vi "Configure Power Analysis (Modulation).vi"(8 "error in (no error)":errorcluster, 9 "Measurement Type (4: Frequency)":i32(ring)=4 items=["Vaverage", "Acrms", "Vratio", "Period", "Frequency", "Pwidth", "Nwidth", "Duty Cycle", "Rise Time", "Fall Time"], 10 "Source (0: V)":i32(ring) items=["V", "I"], 11 "VISA resource name":refnum<visa-resource-name>) -> (0 "error out":errorcluster, 3 "VISA resource name out":refnum<visa-resource-name>)   [LabVIEW 2016, in "Agilent 2000 3000 X-Series.lvlib"]
doc: "Applies a specific modulation analysis type.\n\n<B>Note(s):</B>\nThe Modulation analysis measures the control pulse signal to a switching device (MOSFET) and observes the trending of the pulse width, duty cycle, period, frequency, etc. of the control pulse signal.\n\nUse <B>Read Measurement (Static).vi</B> to read the result of this power analysis."
uses:
  Agilent 2000 3000 X-Series.lvlib
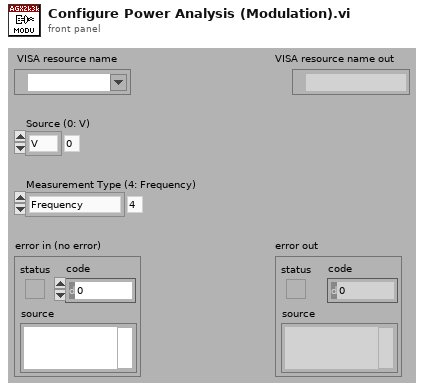
[diagram p1: front panel]
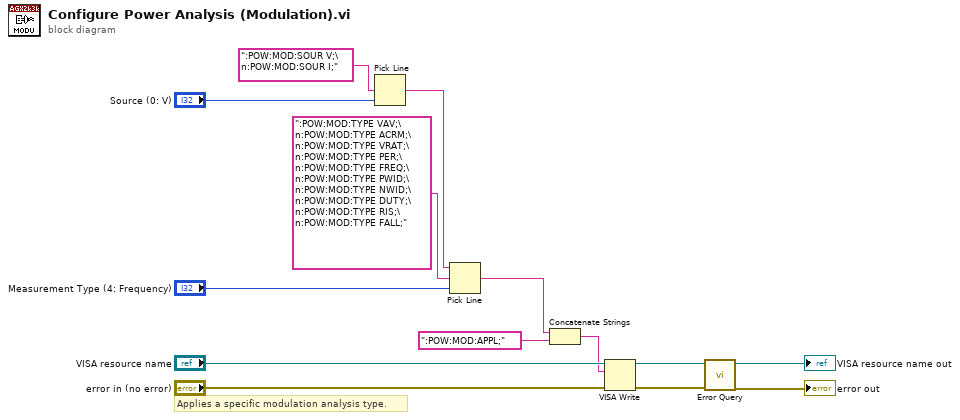
[diagram p0: block diagram]
diagram:
  # "Applies a specific modulation analysis type."
  n1 = Pick Line(multi-line string=":POW:MOD:SOUR V;\n:POW:MOD:SOUR I;", line index="Source (0: V)") -> (output string=w1:string)  [unwired: 1 out]
  n2 = Pick Line(string ("")=w1, multi-line string=":POW:MOD:TYPE VAV;\n:POW:MOD:TYPE ACRM;\n:POW:MOD:TYPE VRAT;\n:POW:MOD:TYPE PER;\n:POW:MOD:TYPE FREQ;\n:POW:MOD:TYPE PWID;\n:POW:MOD:TYPE NWID;\n:POW:MOD:TYPE DUTY;\n:POW:MOD:TYPE RIS;\n:POW:MOD:TYPE FALL;", line index="Measurement Type (4: Frequency)") -> (output string=w3:string)
  n3 = Concatenate Strings(w3, ":POW:MOD:APPL;") -> (w2:string)
  n4 = VISA Write(VISA resource name="VISA resource name", write buffer=w2, error in (no error)="error in (no error)") -> (VISA resource name out=w8:refnum<visa-resource-name>, error out=w7:errorcluster)  [unwired: 1 out]
  n5 = call "Error Query.vi"("error in (no error)"=w7, "VISA resource name"=w8) -> ("error out"=→"error out":errorcluster, "VISA resource name out"=→"VISA resource name out":refnum<visa-resource-name>)  [unwired: 8 out]
